vi "GetNumberOfItems.vi"(0 "object in":refnum<class "Component.lvclass">, 5 "Error In":errorcluster) -> (14 "object out":refnum<class "Component.lvclass">, 16 "ItemsInside":T1, 19 "Error Out":errorcluster)   [LabVIEW 2024, in "Component.lvclass"]
uses:
  Component.lvclass
  Items Inside Map.ctl
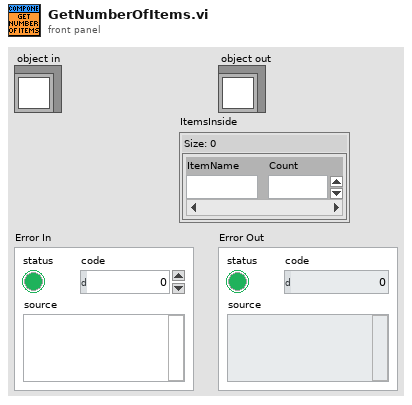
[diagram p1: front panel]
types:
  T1 = typedef "Items Inside Map.ctl" = map{string, u64}
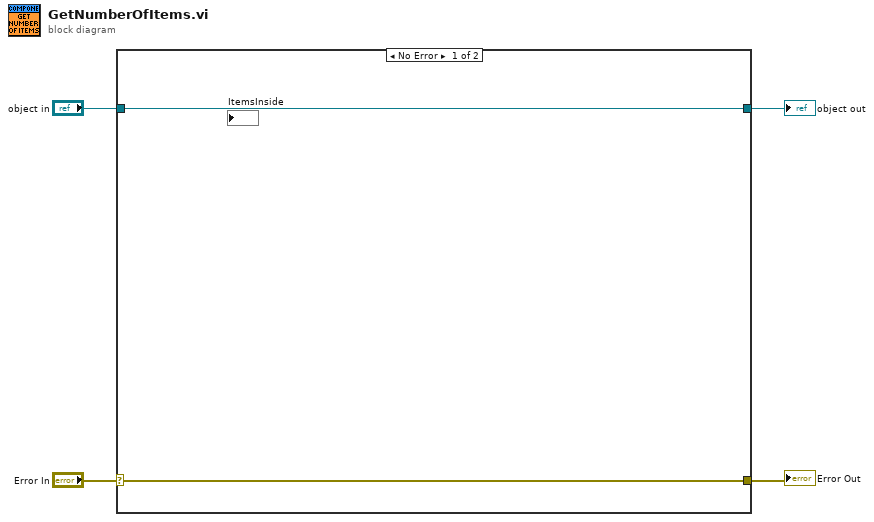
[diagram p0: block diagram]
diagram:
  n1 = case shown="No Error" "Error In" {
    selector: "Error In" -> [w6 w8]
    tunnel: [w6 w8] -> w3
    tunnel: [w5 w7] -> w1
    tunnel: "object in" -> [w5 w7]
    frame No Error {
    }
    frame Error {
    }
  }
  "Error Out" <- w3
  "object out" <- w1
